vi "Bounds.vi"(1 "XRef":refnum<vi>, 2 "State In":T2) -> (0 "Bounds":cluster{"Width":T1, "Height":T1})   [LabVIEW 2018, in "OpenG Conditiional Auto-Indexing Tunnel.xnode"]
uses:
  OpenG Conditiional Auto-Indexing Tunnel.xnode
  State.ctl
  <vilib>/XNodeSupport/XNodeInt.ctl
  <vilib>/XNodeSupport/NI_XNodeSupport.lvlib
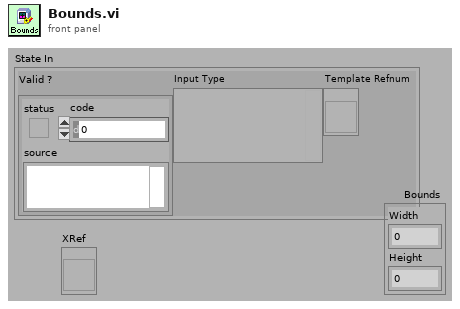
[diagram p1: front panel]
types:
  T1 = typedef "NI_XNodeSupport.lvlib/XNodeInt.ctl" = i32
  T2 = typedef "OpenG Conditiional Auto-Indexing Tunnel.xnode/State.ctl" = cluster{"Valid ?":errorcluster, "Input Type":variant, "Template Refnum":refnum<vi>}
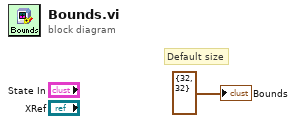
[diagram p0: block diagram]
diagram:
  # "Default size"
  "Bounds" <- cluster{"Width":T1, "Height":T1} {"Width"=32, "Height"=32} ("Bounds")
